vi "Arduino Debug Program - test exhaustive.vi"() -> ()   [LabVIEW 2021]
uses:
  Debug Program Settings.ctl
  Filter Wheel Arduino Homing cluster.ctl
  fb3a7510-300d-4356-a606-047e378fbe38.vi
  a587f9ad-3700-458a-b8a5-e2108659c085.vi
  FW Arduino Control.lvclass
panel:
  out "Plot res":dbl[][](graph)
  out "Responses history 2D out 2":string[][](array[string])=[["[Command Recv(18)]", "Motor ID     :", "State        :", "Direction    :", "Switch       :", "# of steps   :", "Step max rate:", "Ramp Slope   :", "# of position:", "com_success", "Q1S", "EOR1:"]]
  in  "Stop cycle?":bool
  in  "New file?":bool
  in  "Log file path":path=path "C:/Users/gsfcprime/Documents/Logs/FW_test-logs"
  out "Run time":dbl
  out "Currt  time":timestamp
  out "Stopped?":bool
  out "String":string
  in  "Number of moves":u16
  out "cycle  time":dbl
  out "start time":timestamp
  out "End time":timestamp
  in  "milliseconds to wait":u32
  out "Last report saved in:":path
  in  "report file path":path=path "C:/Users/gsfcprime/Documents/PRIME_documentation/Reports"
  in  "Generate report":bool
  out "Sw q response":string
  in  "tail offset:":i32=12
  in  "Reset history":bool
  out "Responses history 2D out":string[][](array[string])
  in  "Homing Parameters":T1={"Direction (F: CW)"=TRUE, "Speed"=150, "Accel"=400, "Min Distance"=2800, "Short Leg"=900}
  out "Move Distance":i32
  out "Moving":bool
  in  "Clear History":bool
  in  "Defaults":T2={"VISA resource name"="COM7", "Speed"=200, "Ramp Slope"=5000, "Motor ID (0:n-1)"=0, "baud rate"=115200}
  in  "Close":bool
  out "Arduino Responses":string
  out "Last Command":string
  in  "Command":string
  in  "Send":bool
  in  "Home Button":bool
  in  "Move":bool
  in  "Counts to Move":i32=2850
  # "Commanding"
  # "Home speed max 200\nor the indentations\nmay be missed."
  # "*  Check communications:\n *      [C]|[check code]|[EOT]\n *\n *  Move:\n *      [M]|Motor # [0-3]|Motor State [1]|Motor Direction [+,-]|Type of Move [R,S]|# Steps [uint]|Delimiter [:]|Max. Rate [uint]|Delimiter [:]|Ramp Slope [uint]|Delimiter [:] (optional)|# Positions [uint] (optional)|[EOT]\n *          * type of move: R --> relative move, S --> switch move\n *          * if number of steps is 0 --> free run\n *          * if Ramp Slope == 0 -> no ramp (start at max. rate)\n *          * may specify the number of position to move for a switch move.  if not specified, defaults to 1 position.\n *\n *  Emergency Stop:\n *      [M]|Motor # [0-3]|Motor State [0]|[EOT]\n *\n *  Get Motor Completed Steps:\n *      [Q]|Motor # [0-3]|[C]|[EOT]\n *  Get Motor Direction:\n *      [Q]|Motor # [0-3]|[D]|[EOT]\n *  Get Motor Step Rate:\n *      [Q]|Motor # [0-3]|[R]|[EOT]\n *  Get Switch State:\n *      [Q]|Motor # [0-3]|[S]|[EOT]\n *\n *  Set Emergency Ramp Multiplier:\n *      [V]|Motor # [0-3]|[E]|Multiplier [uint]|[EOT]\n */"
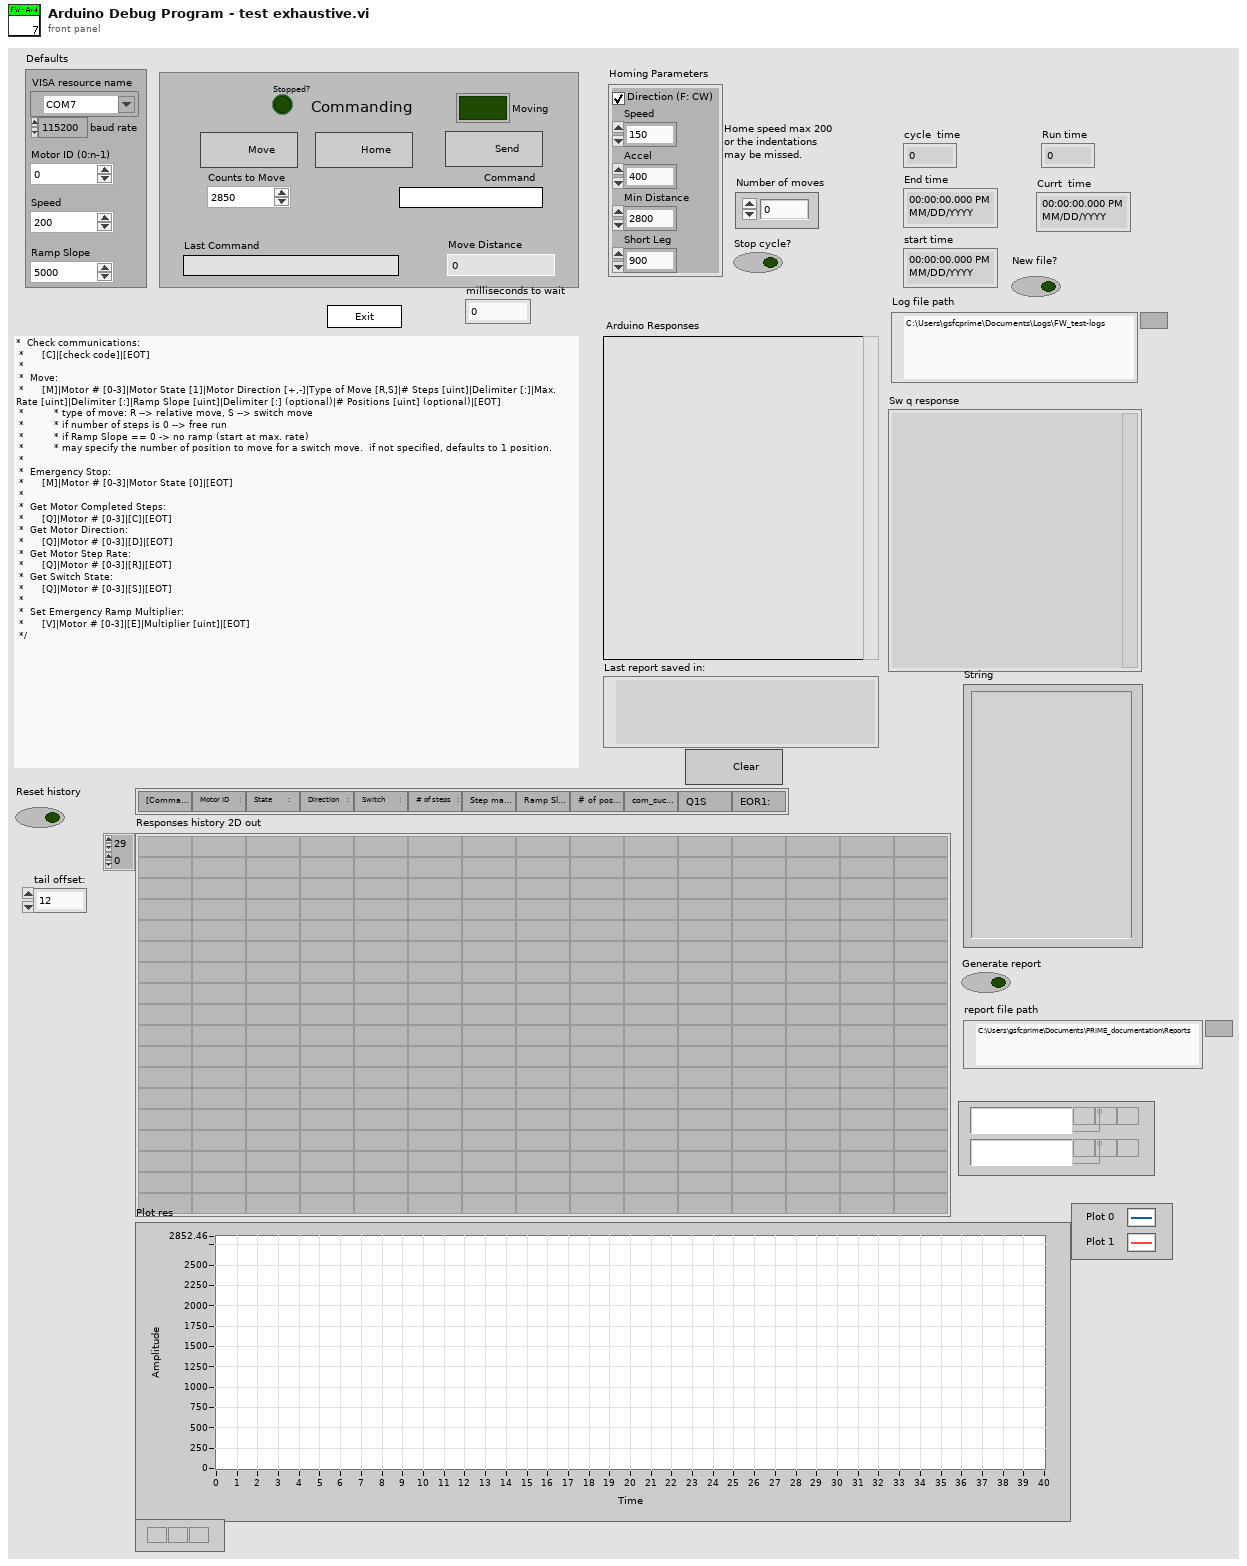
[diagram p1: front panel]
types:
  T1 = typedef "Filter Wheel Arduino Homing cluster.ctl" = cluster{"Direction (F: CW)":bool, "Speed":i32, "Accel":i32, "Min Distance":i32, "Short Leg":i32}
  T2 = typedef "Debug Program Settings.ctl" = cluster{"VISA resource name":refnum<visa-resource-name>, "Speed":i32, "Ramp Slope":i32, "Motor ID (0:n-1)":i32, "baud rate":u32}
  T3 = cluster{"state":refnum<user-event>, "Defaults":T2, "cmd string":string, "connected":bool, "Moving":bool, "log ref":refnum<file>}
  T4 = enum32{"invalid app kind", "Development System", "Run Time System", "Student Edition", "Embedded LabVIEW", "Evaluation", "Custom"}
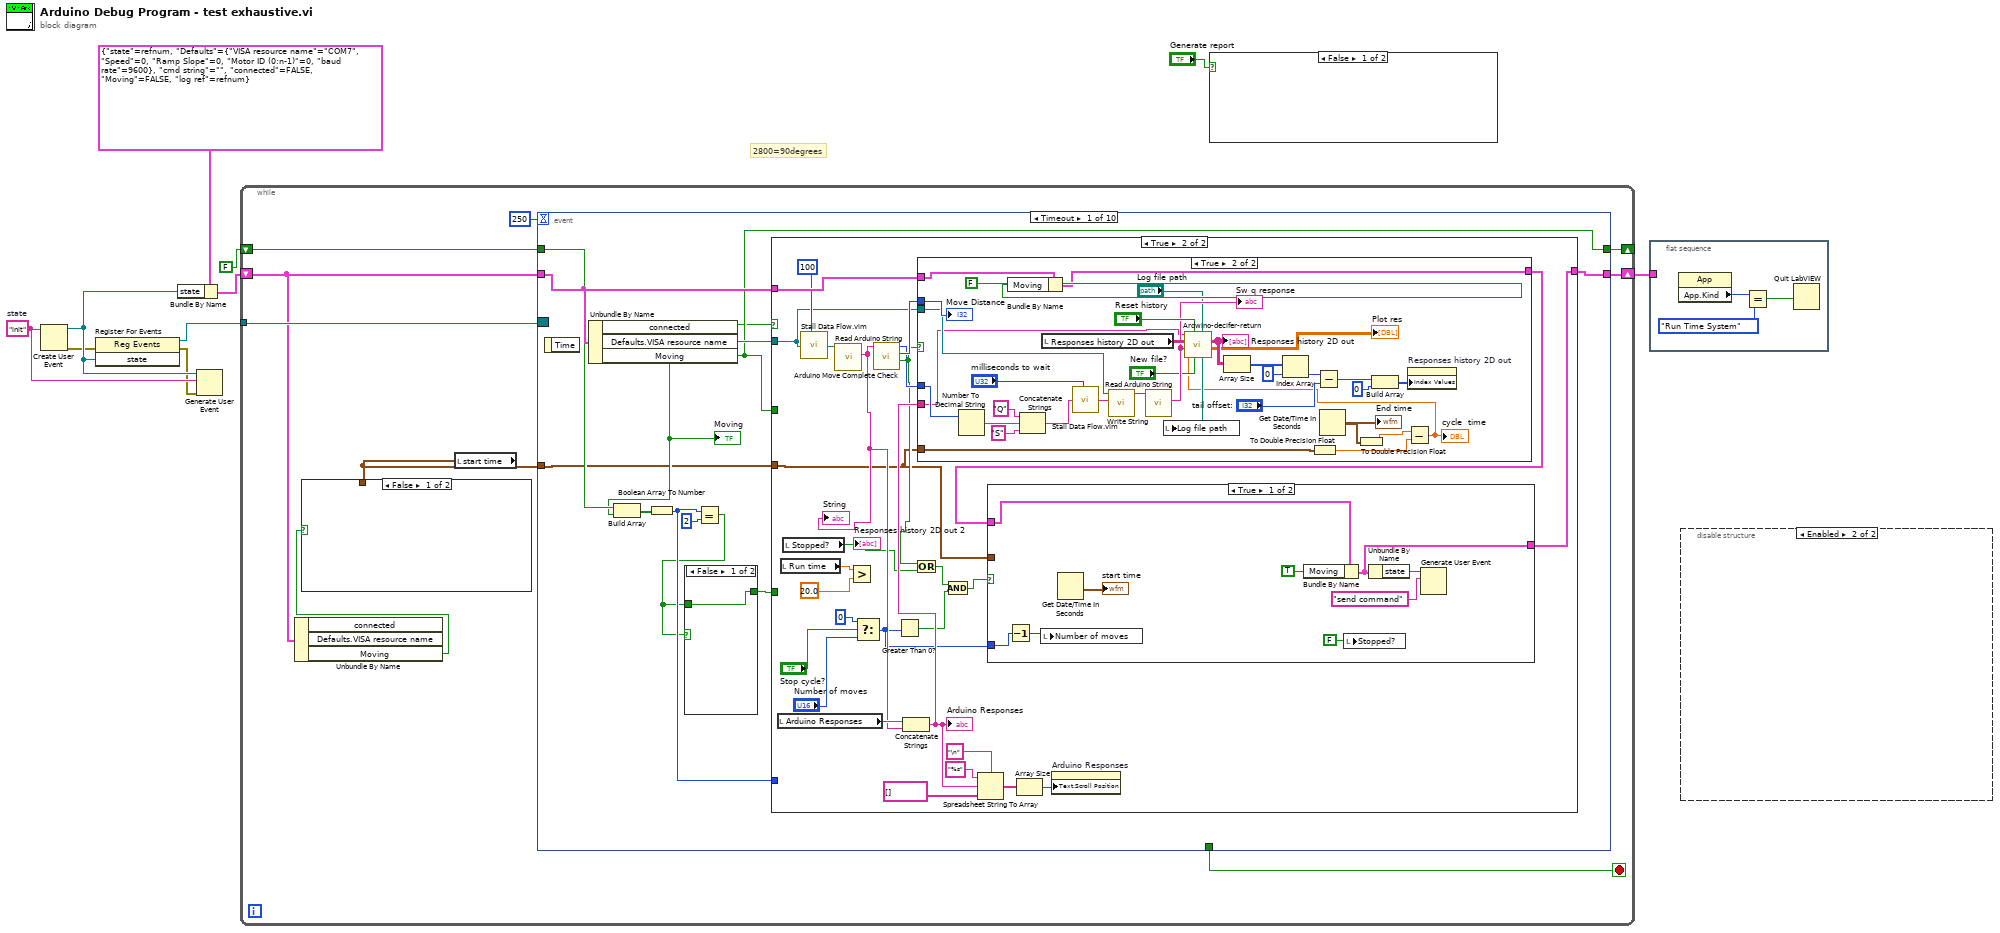
[diagram p0: block diagram]
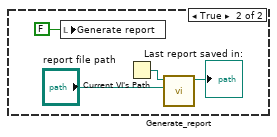
[diagram p2: hidden frame]
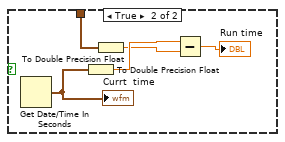
[diagram p4: hidden frame]
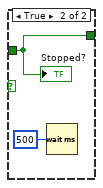
[diagram p5: hidden frame]
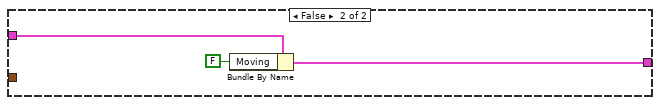
[diagram p7: hidden frame]
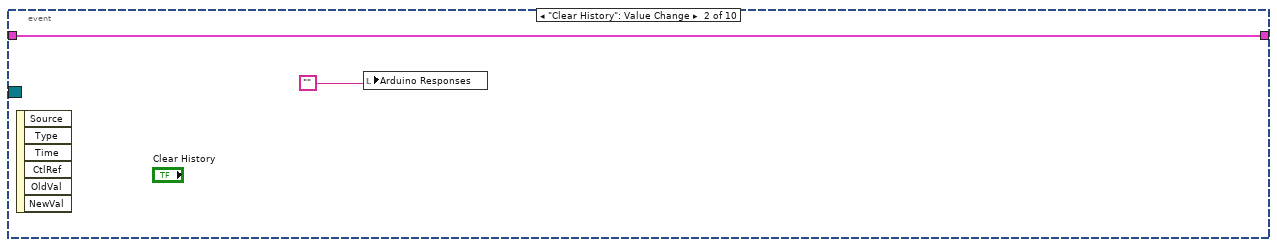
[diagram p9: hidden frame]
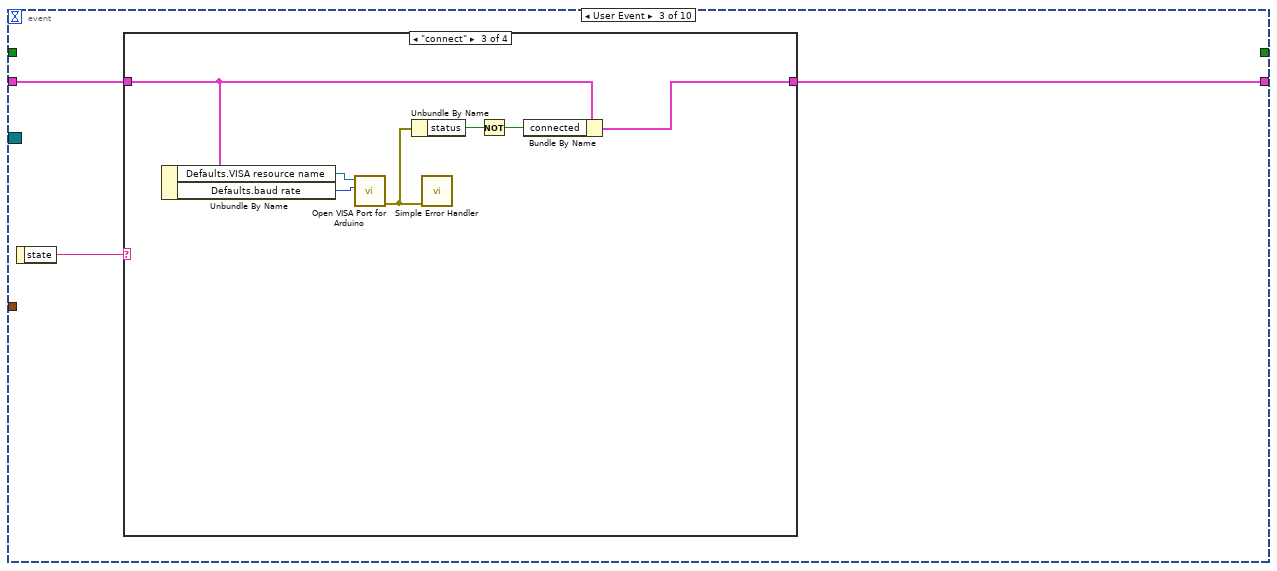
[diagram p10: hidden frame]
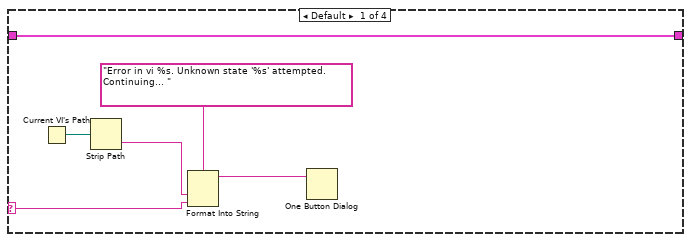
[diagram p11: hidden frame]
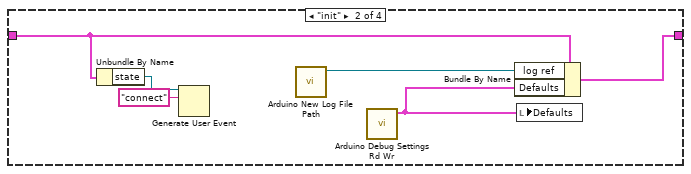
[diagram p12: hidden frame]
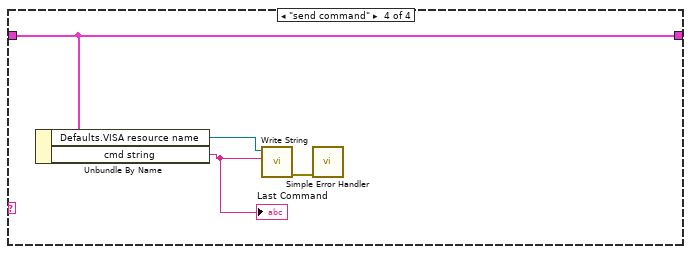
[diagram p13: hidden frame]
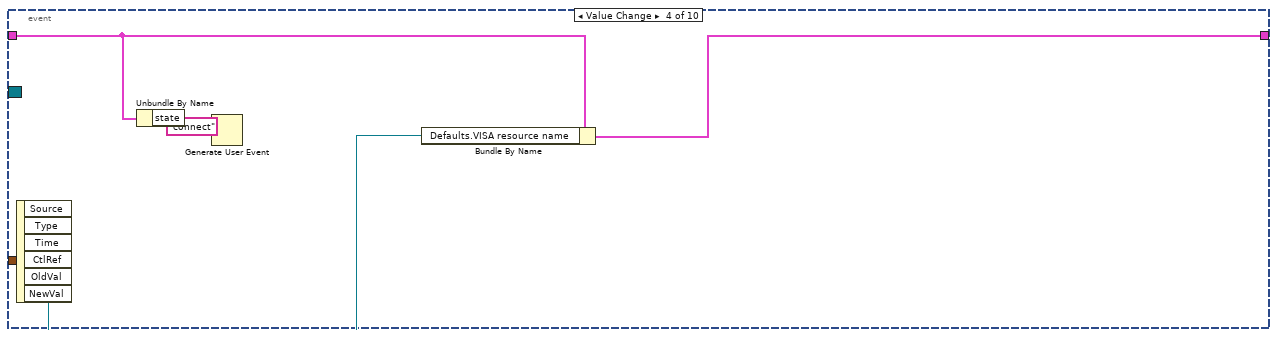
[diagram p14: hidden frame]
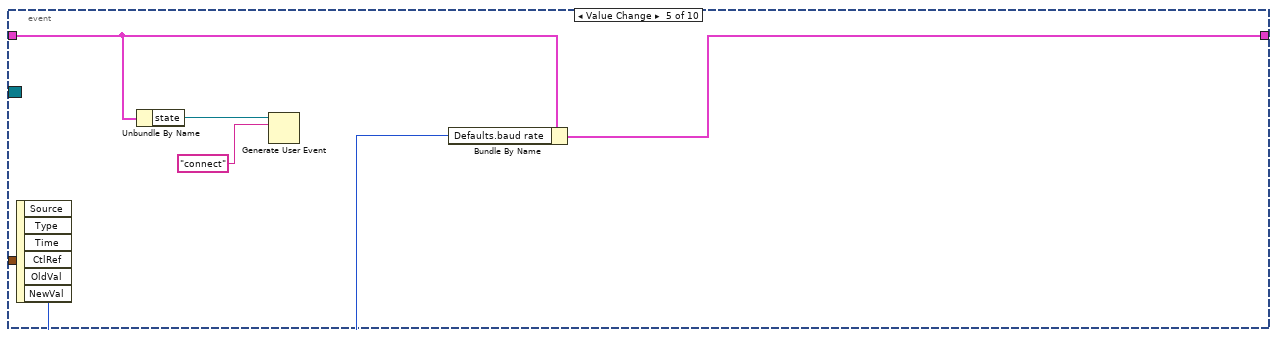
[diagram p15: hidden frame]
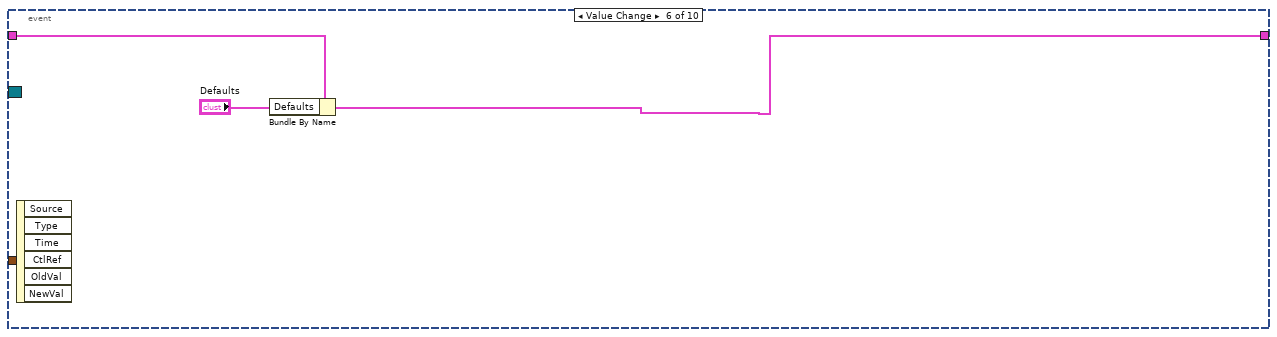
[diagram p16: hidden frame]
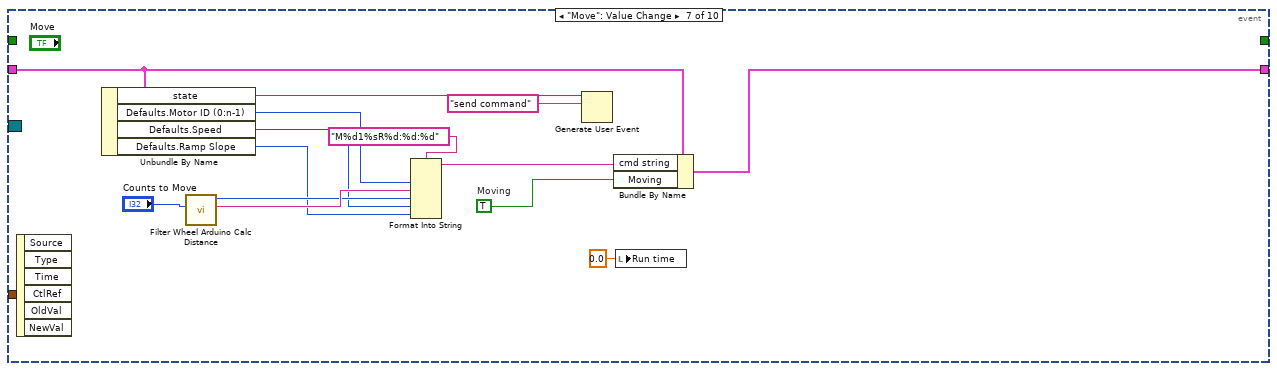
[diagram p17: hidden frame]
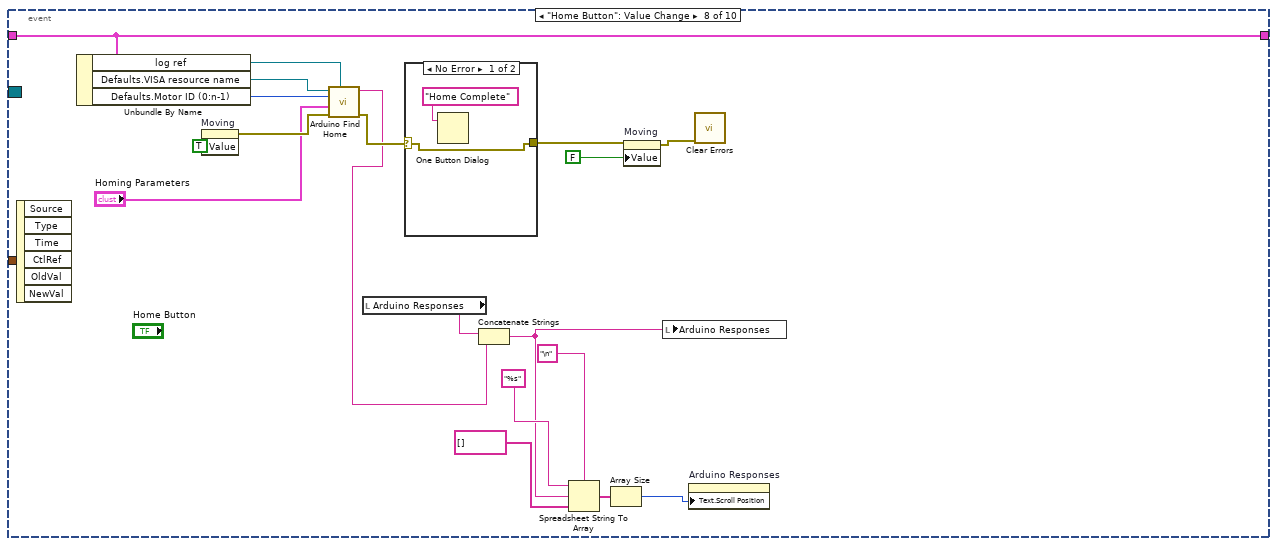
[diagram p18: hidden frame]
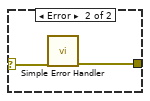
[diagram p19: hidden frame]
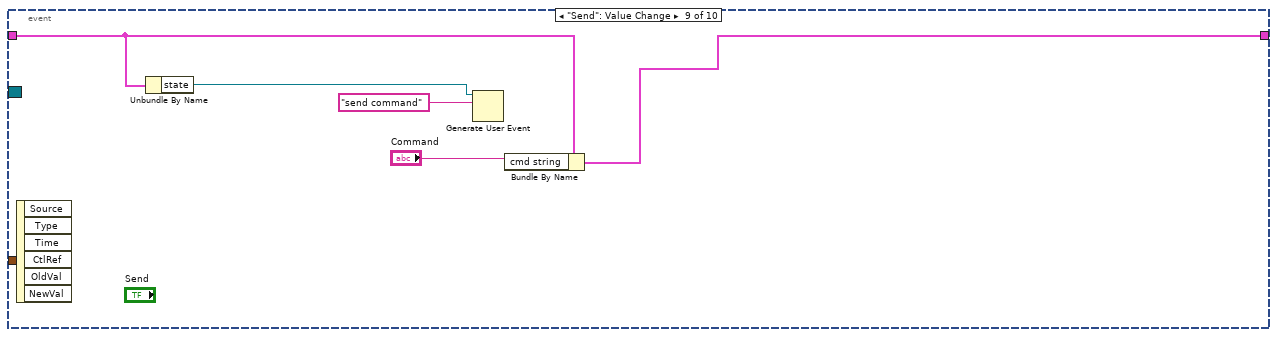
[diagram p20: hidden frame]
diagram:
  w6 = "init"  # state
  # "2800=90degrees"
  n1 = Create User Event(user event datatype=w6) -> (user event=w8:refnum<user-event>, error out=w4:errorcluster)  [unwired: 1 in]
  n2 = register-events(error in=w4, w8) -> (reference out=w7:refnum<event-registration>, error out=w5:errorcluster)  [unwired: 1 in]
  n3 = Bundle By Name(cluster=T3 {"state"=refnum, "Defaults"={"VISA resource name"="COM7", "Speed"=0, "Ramp Slope"=0, "Motor ID (0:n-1)"=0, "baud rate"=9600}, "cmd string"="", "connected"=FALSE, "Moving"=FALSE, "log ref"=refnum}, "state"=w8) -> (w9:T3)
  n4 = Generate User Event(user event=w8, event data cluster=w6, error in=w5) -> ()  [unwired: 1 in, 2 out]
  n5 = while {
    tunnel: w7 -> [w19]
    shift-right: [w18] -> w3
    shift-left: w9 -> [w12]
    shift-right: [w15] -> _
    shift-left: FALSE ("Moving") -> [w14]
    stop <- w17 stop-if-true
    n6 = Unbundle By Name(w12) -> ("Moving"=w11:bool)  [unwired: 2 out]
    n7 = local read "start time"() -> (w13:timestamp)
    n8 = case shown="False" w11 {
      tunnel: w13 -> [_ w24]
      frame False {
      }
      frame True {
        n9 = Get Date/Time In Seconds() -> (seconds since 1Jan1904=w23:timestamp)
        "Currt  time" <- w23
        n10 = To Double Precision Float(number=w23) -> (double precision float=w22:dbl)
        n11 = To Double Precision Float(number=w24) -> (double precision float=w21:dbl)
        n12 = Subtract(x=w22, y=w21) -> (x-y=→"Run time":dbl)
      }
    }
    n13 = event shown="[0] Timeout" {
      selector: w19 -> [_ _ _ _ _ _ _ _ _ _]
      dyn-events: _ -> [_ _ _ _ _ _ _ _ _ _]
      timeout: 250 -> [_ _ _ _ _ _ _ _ _ _]
      tunnel: w12 -> [w34 w117 w119 w144 w149 w156 w163 w185 w196 w202]
      tunnel: [w35 w117 w118 w145 w150 w154 w159 w185 w197 w202] -> w18
      tunnel: [_ _ _ _ _ _ _ _ _ "Close"] -> w17
      tunnel: [w29 _ _ _ _ _ _ _ _ _] -> w15
      tunnel: w14 -> [w33 _ _ _ _ _ _ _ _ _]
      tunnel: w13 -> [w25 _ _ _ _ _ _ _ _ _]
      event Timeout {
        n14 = event-data() -> ()  [unwired: 1 in, 1 out]
        n15 = Unbundle By Name(w34) -> ("connected"=w28:bool, "Defaults.VISA resource name"=w36:refnum<visa-resource-name>, "Moving"=w29:bool)
        "Moving" <- w29
        n16 = Build Array(w33, w29) -> (w32:bool[])
        n17 = Boolean Array To Number(Boolean array=w32) -> (number=w30:u32)
        n18 = Equal?(x=w30, y=u32 2) -> (x = y?=w27:bool)
        n19 = case shown="False" w27 {
          tunnel: w27 -> [w37 w38]
          tunnel: [w37 w38] -> w26
          frame False {
          }
          frame True {
            n20 = Wait (ms)(milliseconds to wait=u32 500) -> ()  [unwired: 1 out]
            "Stopped?" <- w38
          }
        }
        n21 = case shown="True" w28 {
          tunnel: w36 -> [_ w56]
          tunnel: w29 -> [_ _]
          tunnel: w34 -> [w40 w62]
          tunnel: [w40 w48] -> w35
          tunnel: w30 -> [_ _]
          tunnel: w26 -> [_ _]
          tunnel: w25 -> [_ w46]
          frame False {
          }
          frame True {
            n22 = local read "Arduino Responses"() -> (w68:string)
            n23 = local read "Run time"() -> (w54:dbl)
            n24 = local read "Stopped?"() -> (w47:bool)
            n25 = call "Stall Data Flow.vim"("value in"=w56, "milliseconds to wait"=u32 100) -> ("value out"=w57:refnum<visa-resource-name>)  [unwired: 1 out]
            n26 = call "Read Arduino String.vi"("reference"=w57) -> ("response"=w55:string)  [unwired: 8 in, 2 out]
            "String" <- w55
            n27 = Greater?(x=w54, y=20.0) -> ()  [unwired: 1 out]
            n28 = Select(t=u8 0, s="Stop cycle?", f="Number of moves") -> (s? t:f=w41:u16)
            n29 = call "Arduino Move Complete Check.vi"("input string"=w55) -> ("Complete?"=w53:bool, "position"=w61:i32, "m"=w60:i32)  [unwired: 8 in]
            n30 = Greater Than 0?(x=w41) -> (x > 0?=w50:bool)
            n31 = Concatenate Strings(w68, w55) -> (w59:string)
            "Arduino Responses" <- w59
            n32 = Or(x=w53, y=w47) -> (x .or. y?=w51:bool)
            n33 = case shown="True" w53 {
              tunnel: w62 -> [w81 w115]
              tunnel: w61 -> [_ w113]
              tunnel: [w81 w91] -> w49
              tunnel: w56 -> [_ w109]
              tunnel: w60 -> [_ w95]
              tunnel: w59 -> [_ w92]
              tunnel: w46 -> [_ w87]
              frame False {
              }
              frame True {
                n34 = Number To Decimal String(number=w95) -> (decimal integer string=w94:string)  [unwired: 1 in]
                n35 = Bundle By Name(cluster=w115, "Moving"=FALSE) -> (w91:T3)
                n36 = Concatenate Strings("Q", w94, "S") -> (w108:string)
                n37 = local read "Responses history 2D out"() -> (w99:string[][])
                n38 = call "Stall Data Flow.vim"("value in"=w108, "milliseconds to wait"="milliseconds to wait") -> ("value out"=w107:string)  [unwired: 1 out]
                n39 = call "Write String.vi"("String"=w107, "VISA resource name"=w109) -> ("VISA resource name out"=w112:refnum<visa-resource-name>)  [unwired: 8 in, 1 out]
                n40 = call "Read Arduino String.vi"("reference"=w112) -> ("response"=w93:string)  [unwired: 8 in, 2 out]
                "Sw q response" <- w93
                n41 = To Double Precision Float(number=w87) -> (double precision float=w89:dbl)
                n42 = Get Date/Time In Seconds() -> (seconds since 1Jan1904=w88:timestamp)
                "End time" <- w88
                n43 = To Double Precision Float(number=w88) -> (double precision float=w90:dbl)
                n44 = Subtract(x=w90, y=w89) -> (x-y=w83:dbl)
                "cycle  time" <- w83
                n45 = call "Ardwino-decifer-return.vi"("Log file path"="Log file path", "New file?"="New file?", "Reset history"="Reset history", "cycle  time"=w83, "Switch query response"=w93, "Responses history 2D in"=w99, "Arduino Response"=w92) -> ("Waveform Graph"=→"Plot res":dbl[][], "Responses history 2D out"=w100:string[][], "Log file out"=w85:path)  [unwired: 1 in, 1 out]
                "Responses history 2D out" <- w100
                n46 = local write "Log file path"(w85) -> ()
                n47 = Array Size(array=w100) -> (size(s)=w101:i32[])
                n48 = Index Array(array=w101, index=0) -> (element=w103:i32)
                n49 = Subtract(x=w103, y="tail offset:") -> (x-y=w105:i32)
                n50 = Build Array(w105, 0 ("element")) -> (w102:i32[])
                n51 = property on="Responses history 2D out" class="Arr (strict)"("Index Values"=w102) -> ()  [unwired: 2 in, 2 out]
                "Move Distance" <- w113
              }
            }
            n52 = And(x=w51, y=w50) -> (x .and. y?=w52:bool)
            n53 = Spreadsheet String To Array(delimiter (Tab)="\n", format string="%s", spreadsheet string=w59, array type (2D Dbl)=string[] []) -> (array=w65:string[])
            n54 = case shown="True" w52 {
              tunnel: w46 -> [_ _]
              tunnel: w41 -> [w74 _]
              tunnel: w49 -> [w73 w79]
              tunnel: [w72 w78] -> w48
              frame True {
                n55 = Decrement(x=w74) -> (x-1=w77:u16)
                n56 = local write "Number of moves"(w77) -> ()
                n57 = Get Date/Time In Seconds() -> (seconds since 1Jan1904=→"start time":timestamp)
                n58 = Bundle By Name(cluster=w73, "Moving"=TRUE) -> (w72:T3)
                n59 = local write "Stopped?"(FALSE ("Stopped?")) -> ()
                n60 = Unbundle By Name(w72) -> ("state"=w71:refnum<user-event>)
                n61 = Generate User Event(user event=w71, event data cluster="send command" ("event data")) -> ()  [unwired: 2 in, 2 out]
              }
              frame False {
                n62 = Bundle By Name(cluster=w79, "Moving"=FALSE) -> (w78:T3)
              }
            }
            n63 = Array Size(array=w65) -> (size(s)=w63:i32)
            n64 = property on="Arduino Responses" class="Str"("Text.Scroll Position"=w63) -> ()  [unwired: 2 in, 2 out]
          }
        }
      }
      event "Clear History": Value Change {
        n65 = event-data() -> ()  [unwired: 1 in, 6 out]
        n66 = local write "Arduino Responses"("") -> ()
      }
      event User Event {
        n67 = event-data() -> ("state"=w120:string)  [unwired: 1 in]
        n68 = case shown="\"connect\"" w120 {
          selector: w120 -> [w125 _ _ _]
          tunnel: w119 -> [w121 w130 w134 w143]
          tunnel: [w121 w131 w135 w143] -> w118
          frame Default {
            n69 = Current VI's Path() -> (path=w124:path)
            n70 = Strip Path(path=w124) -> (name=w123:string)  [unwired: 1 out]
            n71 = Format Into String(format string="Error in vi %s. Unknown state '%s' attempted. Continuing... ", w123, w125) -> (resulting string=w122:string)  [unwired: 2 in, 1 out]
            n72 = One Button Dialog(message=w122) -> ()  [unwired: 1 in, 1 out]
          }
          frame "init" {
            n73 = Unbundle By Name(w130) -> ("state"=w129:refnum<user-event>)
            n74 = Generate User Event(user event=w129, event data cluster="connect" ("event data")) -> ()  [unwired: 2 in, 2 out]
            n75 = call "Arduino New Log File Path.vi"() -> ("log ref"=w127:refnum<file>)  [unwired: 11 in]
            n76 = call "Arduino Debug Settings Rd Wr.vi"() -> ("Defaults"=w132:T2)  [unwired: 10 in, 1 out]
            n77 = Bundle By Name(cluster=w130, "log ref"=w127, "Defaults"=w132) -> (w131:T3)
            n78 = local write "Defaults"(w132) -> ()
          }
          frame "connect" {
            n79 = Unbundle By Name(w134) -> ("Defaults.VISA resource name"=w139:refnum<visa-resource-name>, "Defaults.baud rate"=w133:u32)
            n80 = call "Open VISA Port for Arduino.vi"("baud rate (9600)"=w133, "VISA resource name"=w139) -> ("error out"=w138:errorcluster)  [unwired: 8 in, 1 out]
            n81 = Unbundle By Name(w138) -> ("status"=w137:bool)
            n82 = call <vilib>:"Simple Error Handler.vi"("error in (no error)"=w138) -> ()  [unwired: 4 in, 5 out]
            n83 = Not(x=w137) -> (.not. x?=w136:bool)
            n84 = Bundle By Name(cluster=w134, "connected"=w136) -> (w135:T3)
          }
          frame "send command" {
            n85 = Unbundle By Name(w143) -> ("Defaults.VISA resource name"=w142:refnum<visa-resource-name>, "cmd string"=w141:string)
            "Last Command" <- w141
            n86 = call "Write String.vi"("String"=w141, "VISA resource name"=w142) -> ("error out"=w140:errorcluster)  [unwired: 8 in, 1 out]
            n87 = call <vilib>:"Simple Error Handler.vi"("error in (no error)"=w140) -> ()  [unwired: 4 in, 5 out]
          }
        }
      }
      event Value Change {
        n88 = event-data() -> ("NewVal"=w146:refnum<visa-resource-name>)  [unwired: 1 in, 5 out]
        n89 = Unbundle By Name(w144) -> ("state"=w148:refnum<user-event>)
        n90 = Generate User Event(user event=w148, event data cluster="connect" ("event data")) -> ()  [unwired: 2 in, 2 out]
        n91 = Bundle By Name(cluster=w144, "Defaults.VISA resource name"=w146) -> (w145:T3)
      }
      event Value Change {
        n92 = event-data() -> ("NewVal"=w151:u32)  [unwired: 1 in, 5 out]
        n93 = Unbundle By Name(w149) -> ("state"=w153:refnum<user-event>)
        n94 = Generate User Event(user event=w153, event data cluster="connect" ("event data")) -> ()  [unwired: 2 in, 2 out]
        n95 = Bundle By Name(cluster=w149, "Defaults.baud rate"=w151) -> (w150:T3)
      }
      event Value Change {
        n96 = event-data() -> ()  [unwired: 1 in, 6 out]
        n97 = Bundle By Name(cluster=w156, "Defaults"="Defaults") -> (w154:T3)
      }
      event "Move": Value Change {
        w160 = TRUE  # Moving
        n98 = event-data() -> ()  [unwired: 1 in, 6 out]
        n99 = Unbundle By Name(w163) -> ("state"=w162:refnum<user-event>, "Defaults.Motor ID (0:n-1)"=w158:i32, "Defaults.Speed"=w166:i32, "Defaults.Ramp Slope"=w165:i32)
        n100 = call "Filter Wheel Arduino Calc Distance.vi"("To Position"="Counts to Move") -> ("Direction"=w168:string, "Counts"=w167:u32)  [unwired: 8 in, 1 out]
        n101 = Format Into String(format string="M%d1%sR%d:%d:%d", w158, w168, w167, w166, w165) -> (resulting string=w164:string)  [unwired: 2 in, 1 out]
        n102 = Generate User Event(user event=w162, event data cluster="send command" ("event data")) -> ()  [unwired: 2 in, 2 out]
        n103 = Bundle By Name(cluster=w163, "cmd string"=w164, "Moving"=w160) -> (w159:T3)
        n104 = local write "Run time"(0.0 ("Run time")) -> ()
      }
      event "Home Button": Value Change {
        n105 = event-data() -> ()  [unwired: 1 in, 6 out]
        n106 = Unbundle By Name(w185) -> ("log ref"=w171:refnum<file>, "Defaults.VISA resource name"=w189:refnum<visa-resource-name>, "Defaults.Motor ID (0:n-1)"=w188:i32)
        n107 = property on="Moving" class="Bool (strict)"("Value"=TRUE ("Moving")) -> (error out=w187:errorcluster)  [unwired: 2 in, 1 out]
        n108 = call "Arduino Find Home.vi"("log ref"=w171, "error in"=w187, "Homing Parameters"="Homing Parameters", "Motor"=w188, "Addr"=w189) -> ("error out"=w184:errorcluster, "Log"=w175:string)  [unwired: 4 in, 1 out]
        n109 = local read "Arduino Responses"() -> (w180:string)
        n110 = case shown="No Error" w184 {
          selector: w184 -> [w190 w193]
          tunnel: [w190 w192] -> w183
          frame No Error {
            n111 = One Button Dialog(message="Home Complete") -> ()  [unwired: 1 in, 1 out]
          }
          frame Error {
            n112 = call <vilib>:"Simple Error Handler.vi"("error in (no error)"=w193) -> ("error out"=w192:errorcluster)  [unwired: 4 in, 4 out]
          }
        }
        n113 = Concatenate Strings(w180, w175) -> (w174:string)
        n114 = Spreadsheet String To Array(delimiter (Tab)="\n", format string="%s", spreadsheet string=w174, array type (2D Dbl)=string[] []) -> (array=w179:string[])
        n115 = Array Size(array=w179) -> (size(s)=w173:i32)
        n116 = property on="Moving" class="Bool (strict)"(error in=w183, "Value"=FALSE ("Moving")) -> (error out=w172:errorcluster)  [unwired: 1 in, 1 out]
        n117 = local write "Arduino Responses"(w174) -> ()
        n118 = property on="Arduino Responses" class="Str"("Text.Scroll Position"=w173) -> ()  [unwired: 2 in, 2 out]
        n119 = call <vilib>:"Clear Errors.vi"("error in (no error)"=w172) -> ()  [unwired: 5 in, 2 out]
      }
      event "Send": Value Change {
        n120 = event-data() -> ()  [unwired: 1 in, 6 out]
        n121 = Unbundle By Name(w196) -> ("state"=w195:refnum<user-event>)
        n122 = Generate User Event(user event=w195, event data cluster="send command" ("event data")) -> ()  [unwired: 2 in, 2 out]
        n123 = Bundle By Name(cluster=w196, "cmd string"="Command") -> (w197:T3)
      }
      event "Close": Value Change {
        n124 = event-data() -> ()  [unwired: 1 in, 6 out]
        n125 = Unbundle By Name(w202) -> ("Defaults.VISA resource name"=w201:refnum<visa-resource-name>, "Defaults"=w200:T2)
        n126 = call "Arduino Debug Settings Rd Wr.vi"("Write? (F:Read)"=TRUE, "Defaults"=w200) -> ()  [unwired: 8 in, 2 out]
        n127 = VISA Close(VISA resource name=w201) -> ()  [unwired: 1 in, 1 out]
      }
    }
  }
  n128 = case shown="False" "Generate report" {
    frame False {
    }
    frame True {
      n129 = local write "Generate report"(FALSE ("Generate report")) -> ()
      n130 = Current VI's Path() -> (path=w207:path)
      n131 = call "Generate_report.vi"("report file path"="report file path", "VI"=w207) -> ("appended path"=→"Last report saved in:":path)  [unwired: 9 in]
    }
  }
  n132 = flat-sequence {
    tunnel: w3 -> [_]
    frame #0 {
      n133 = property class="App"() -> ("App.Kind"=w210:T4)  [unwired: 2 in, 2 out]
      n134 = Equal?(x=w210, y=T4."Run Time System") -> (x = y?=w208:bool)
      n135 = Quit LabVIEW(quit? (T)=w208) -> ()
    }
  }
  n136 = disable-structure shown="Enabled" {
    frame Disabled {
    }
    frame Enabled {
    }
  }
